vi "prendido y apagado del led 8.1.vi"() -> ()   [LabVIEW 2017]
panel:
  out "Boolean":bool
  in  "stop":bool
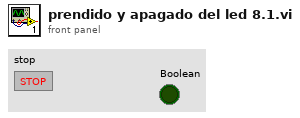
[diagram p1: front panel]
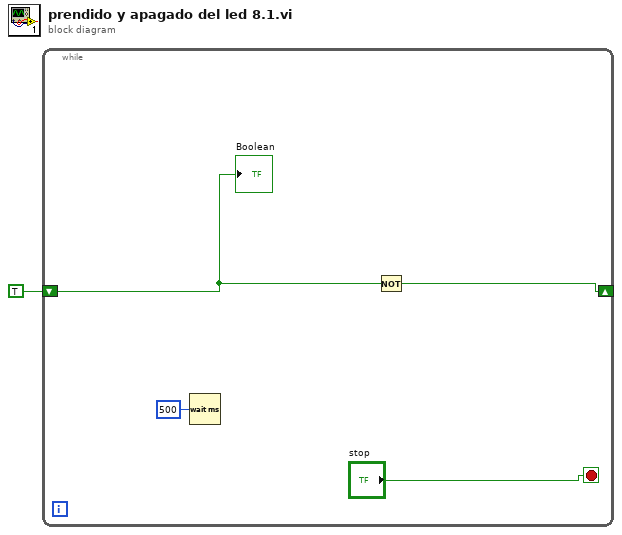
[diagram p0: block diagram]
diagram:
  n1 = while {
    shift-right: [w4] -> _
    shift-left: TRUE -> [w2]
    stop <- "stop" stop-if-true
    n2 = Wait (ms)(milliseconds to wait=u32 500) -> ()  [unwired: 1 out]
    n3 = Not(x=w2) -> (.not. x?=w4:bool)
    "Boolean" <- w2
  }
